vi "Read_RobotLiftOutput.vi"(8 "error in (no error)":errorcluster, 11 "RobotLiftData in":refnum<class "RobotLiftData.lvclass">) -> (0 "error out":errorcluster, 2 "RobotLiftOutput":T1, 3 "RobotLiftData out":refnum<class "RobotLiftData.lvclass">)   [LabVIEW 2017, in "RobotLiftData.lvclass"]
uses:
  RobotLiftData.lvclass
  Team-code/RobotLiftOutput.ctl
  RobotLiftData.lvclass/RobotLiftData.ctl
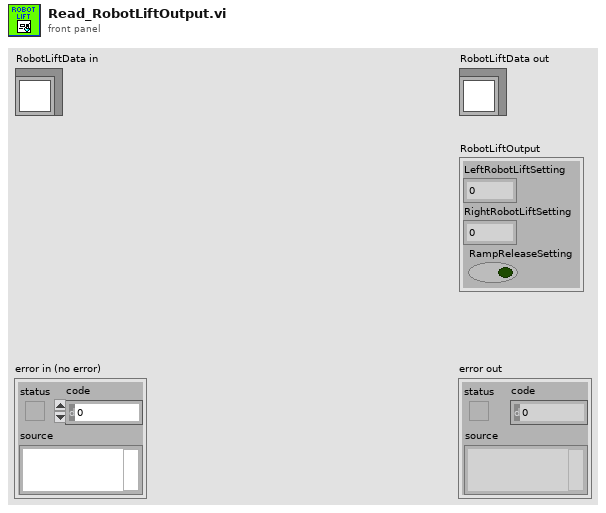
[diagram p1: front panel]
types:
  T1 = typedef "RobotLiftData.lvclass/RobotLiftOutput.ctl" = cluster{"LeftRobotLiftSetting":dbl, "RightRobotLiftSetting":dbl, "RampReleaseSetting":bool}
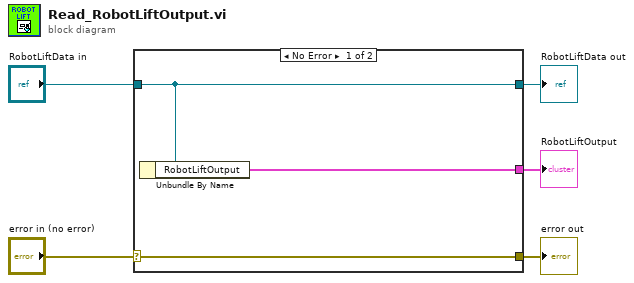
[diagram p0: block diagram]
diagram:
  n1 = case shown="No Error" "error in (no error)" {
    selector: "error in (no error)" -> [w8 w9]
    tunnel: [w8 w9] -> w4
    tunnel: [w7 w10] -> w2
    tunnel: "RobotLiftData in" -> [w7 w10]
    tunnel: [w6 _] -> w1
    frame No Error {
      n2 = Unbundle By Name(w7) -> ("RobotLiftOutput"=w6:T1)
    }
    frame Error {
    }
  }
  "error out" <- w4
  "RobotLiftData out" <- w2
  "RobotLiftOutput" <- w1
